vi "writeSDOI16.vi"(6 "object sub-index (0)":u8 format="%x", 7 "object index":u16 format="%x", 8 "error in (no error)":errorcluster, 9 "interface object in":refnum<k20>, 10 "inputNumber":i16, 11 "MotorController in":refnum<class "MotorController.lvclass">) -> (0 "error out":errorcluster, 1 "interface object out":refnum<k20>, 2 "completion code":u32, 3 "MotorController out":refnum<class "MotorController.lvclass">)   [LabVIEW 2017, in "MotorController.lvclass"]
uses:
  MotorController.lvclass
  MotorController.lvclass/MotorController.ctl
  <vilib>/CANopenLib/CANOPEN.llb/CANopen SDO Create.vi
  <vilib>/CANopenLib/CANOPEN.llb/CANopen SDO Write [I16].vi
  <vilib>/CANopenLib/CANOPEN.llb/CANopen SDO Close.vi
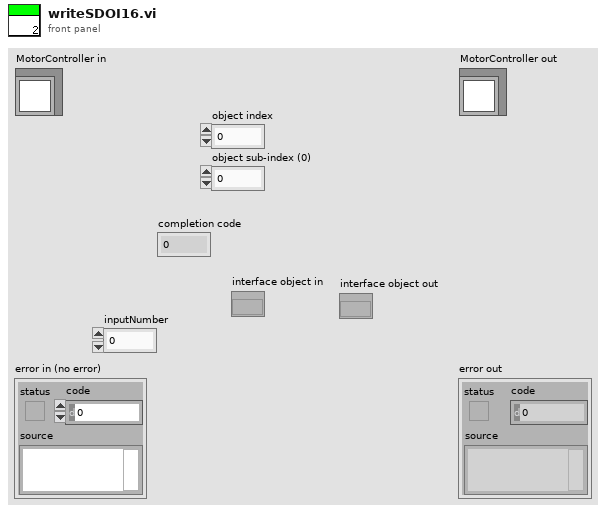
[diagram p1: front panel]
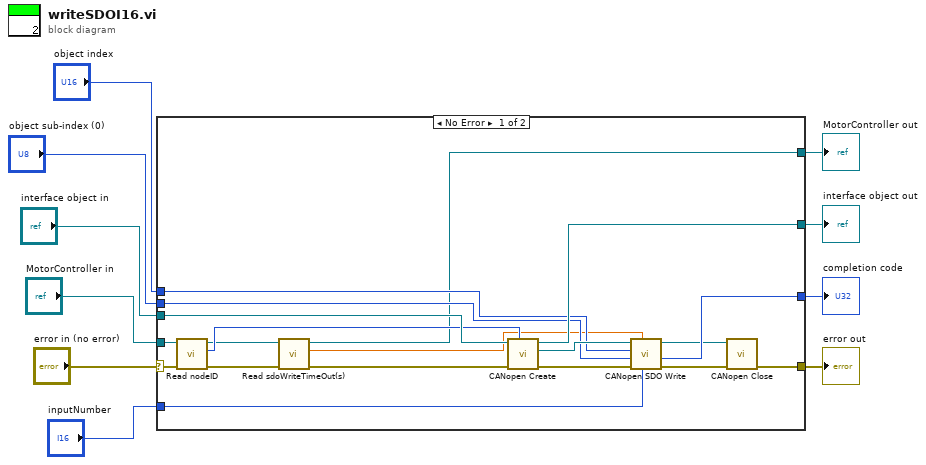
[diagram p0: block diagram]
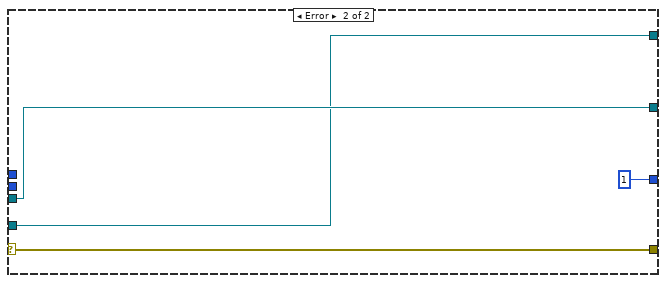
[diagram p2: hidden frame]
diagram:
  n1 = case shown="No Error" "error in (no error)" {
    selector: "error in (no error)" -> [w27 w33]
    tunnel: [w20 w33] -> w1
    tunnel: [w16 w30] -> w7
    tunnel: [w29 w31] -> w8
    tunnel: "interface object in" -> [w28 w31]
    tunnel: "object index" -> [w24 _]
    tunnel: "object sub-index (0)" -> [w23 _]
    tunnel: [w22 u32 1 ("completion code")] -> w3
    tunnel: "MotorController in" -> [w12 w30]
    tunnel: "inputNumber" -> [w11 _]
    frame No Error {
      n2 = call "Read nodeID.vi"("error in (no error)"=w27, "MotorController in"=w12) -> ("error out"=w15:errorcluster, "nodeID"=w26:u8, "MotorController out"=w17:refnum<class "MotorController.lvclass">)  [unwired: 7 in]
      n3 = call "Read sdoWriteTimeOut(s).vi"("error in (no error)"=w15, "MotorController in"=w17) -> ("error out"=w14:errorcluster, "sdoWriteTimeOut(s)"=w18:dbl, "MotorController out"=w16:refnum<class "MotorController.lvclass">)  [unwired: 7 in]
      n4 = call-poly <vilib>:"CANopen Create.vi"("node-ID"=w26, "error in (no error)"=w14, "interface object in"=w28) -> ("error out"=w13:errorcluster, "SDO object out"=w25:refnum<k20>, "interface object out"=w29:refnum<k20>)  [unwired: 6 in]
      n5 = call-poly <vilib>:"CANopen SDO Write.vi"("I16 data"=w11, "timeout (1s)"=w18, "error in (no error)"=w13, "object sub-index (0)"=w23, "object index"=w24, "SDO object in"=w25) -> ("error out"=w21:errorcluster, "completion code"=w22:u32, "SDO object out"=w19:refnum<k20>)  [unwired: 3 in]
      n6 = call-poly <vilib>:"CANopen Close.vi"("error in (no error)"=w21, "SDO object in"=w19) -> ("error out"=w20:errorcluster)  [unwired: 9 in]
    }
    frame Error {
    }
  }
  "error out" <- w1
  "MotorController out" <- w7
  "interface object out" <- w8
  "completion code" <- w3
